vi "HXG2_Gain Schedule Select.vi"(8 "error in (no error)":errorcluster, 10 "SchedLimsArray":cluster{"LL  ":dbl, "UL":dbl}[](array[cluster]), 11 "SP In":dbl) -> (0 "error out":errorcluster, 3 "Schedule":i32)   [LabVIEW 2012]
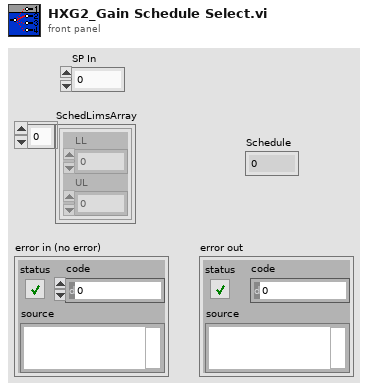
[diagram p1: front panel]
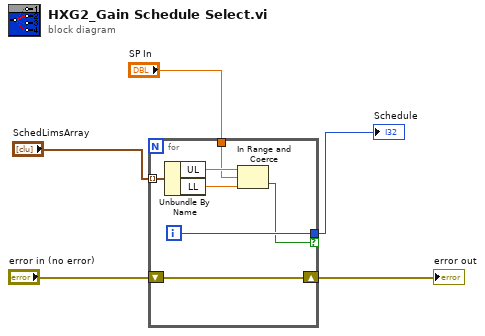
[diagram p0: block diagram]
diagram:
  n1 = for {
    tunnel: "SchedLimsArray" -> [w12] mode=indexing
    tunnel: [w9] -> w2 if=w8
    tunnel: "SP In" -> [w7]
    shift-right: [w6] -> w5
    shift-left: "error in (no error)" -> [w6]
    i -> [w9]
    n2 = Unbundle By Name(w12) -> ("UL"=w11:dbl, "LL"=w10:dbl)
    n3 = In Range and Coerce(upper limit=w11, x=w7, lower limit=w10) -> (In Range?=w8:bool)  [unwired: 1 out]
  }
  "error out" <- w5
  "Schedule" <- w2
